vi "svx_Set Column Header.vi"(0 "result table":string[][](table), 5 "scaled signals [EU]":waveform(dbl)[](array[waveform]), 11 "error in (no error)":errorcluster) -> (4 "dup result table":string[][](table), 6 "column headers":string[](array[string]), 15 "error out":errorcluster)   [LabVIEW 2017]
doc: "Generates a table based on the results of a fractional-octave analysis."
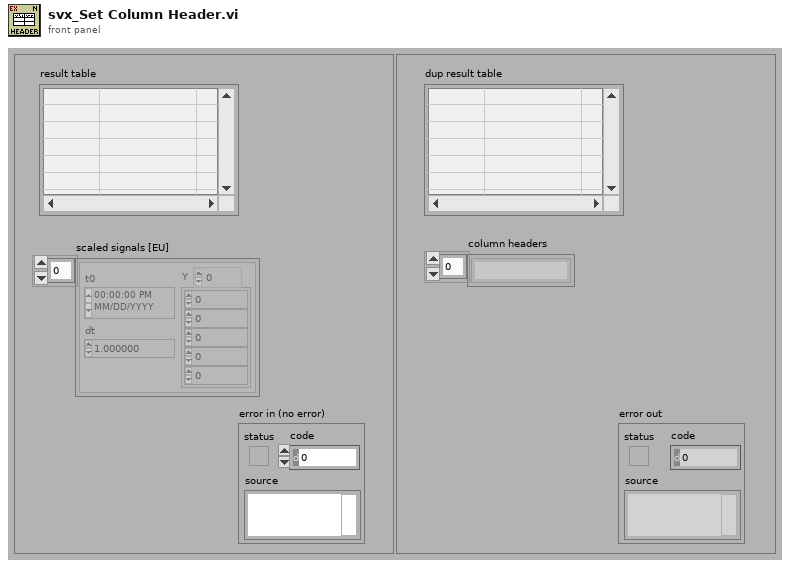
[diagram p1: front panel]
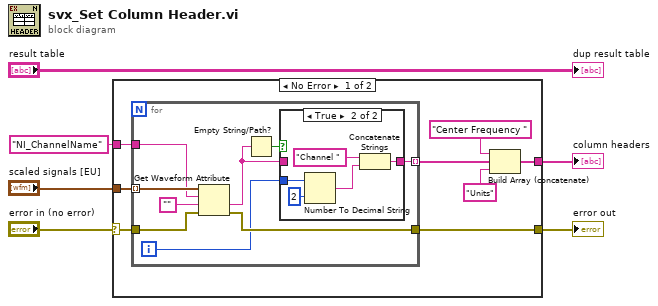
[diagram p0: block diagram]
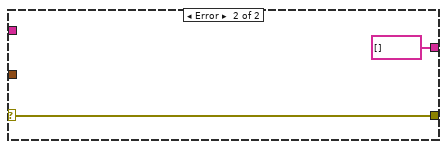
[diagram p3: hidden frame]
diagram:
  n1 = case shown="No Error" "error in (no error)" {
    selector: "error in (no error)" -> [w12 w31]
    tunnel: [w13 w31] -> w3
    tunnel: "scaled signals [EU]" -> [w14 _]
    tunnel: [w9 string[] []] -> w2
    tunnel: "NI_ChannelName" ("name") -> [w7 _]
    frame No Error {
      n2 = for {
        tunnel: w14 -> [w23] mode=indexing
        tunnel: [w21] -> w13
        tunnel: w12 -> [w17]
        tunnel: [w20] -> w11 mode=indexing
        tunnel: w7 -> [w15]
        i -> [w16]
        n3 = Get Waveform Attribute(4:w17, 5:"", 6:w15, 7:w23) -> (0:w21:errorcluster, 1:w19:string)  [unwired: 2 out]
        n4 = Empty String/Path?(string/path=w19) -> (empty?=w18:bool)
        n5 = case shown="True" w18 {
          tunnel: [w24 w28] -> w20
          tunnel: w19 -> [w24 _]
          tunnel: w16 -> [_ w27]
          frame False {
          }
          frame True {
            n6 = Number To Decimal String(number=w27, width (-)=i16 2) -> (decimal integer string=w25:string)
            n7 = Concatenate Strings("Channel " ("name"), w25) -> (w28:string)
          }
        }
      }
      n8 = Build Array (concatenate)("Center Frequency " ("name"), w11, "Units" ("name")) -> (w9:string[])
    }
    frame Error {
    }
  }
  "error out" <- w3
  "column headers" <- w2
  "dup result table" <- "result table"
